vi "Stepper Motor.vi"() -> ()   [LabVIEW 2019]
doc: "The NI ELVIS III Custom FPGA Project template acquires button data from the onboard button and displays the button value on a Boolean indicator."
uses:
  <vilib>/Platform/TimedLoop/XDataNode/timing_clust.ctl
  <vilib>/Platform/TimedLoop/XDataNode/nitl_modes.ctl
  <vilib>/Platform/TimedLoop/XDataNode/wakeup.ctl
  <vilib>/Platform/TimedLoop/XDataNode/XDataNode.xnode
  <vilib>/Platform/TimedLoop/XDataNode/XDNodeRunTimeDep.lvlib
panel:
  in  "Microstep \nQuantization":dbl=100.0 format="%#_13g"
  in  "Step Period (ms)":i64(knob)=100 min=2 max=200 step=1 scale=2.0..200.0
  in  "Microstep Enable":bool
  out "Coil Activation":bool[](array[boolean])
  in  "Coil Activation Pattern":bool[][](array[boolean])
  out "Error Out":errorcluster
  in  "Stop Button":bool
  # "Mechatronic Actuators Board"
  # "Stepper Motor"
  # "A"
  # "B"
  # "C"
  # "D"
  # "A"
  # "B"
  # "C"
  # "D"
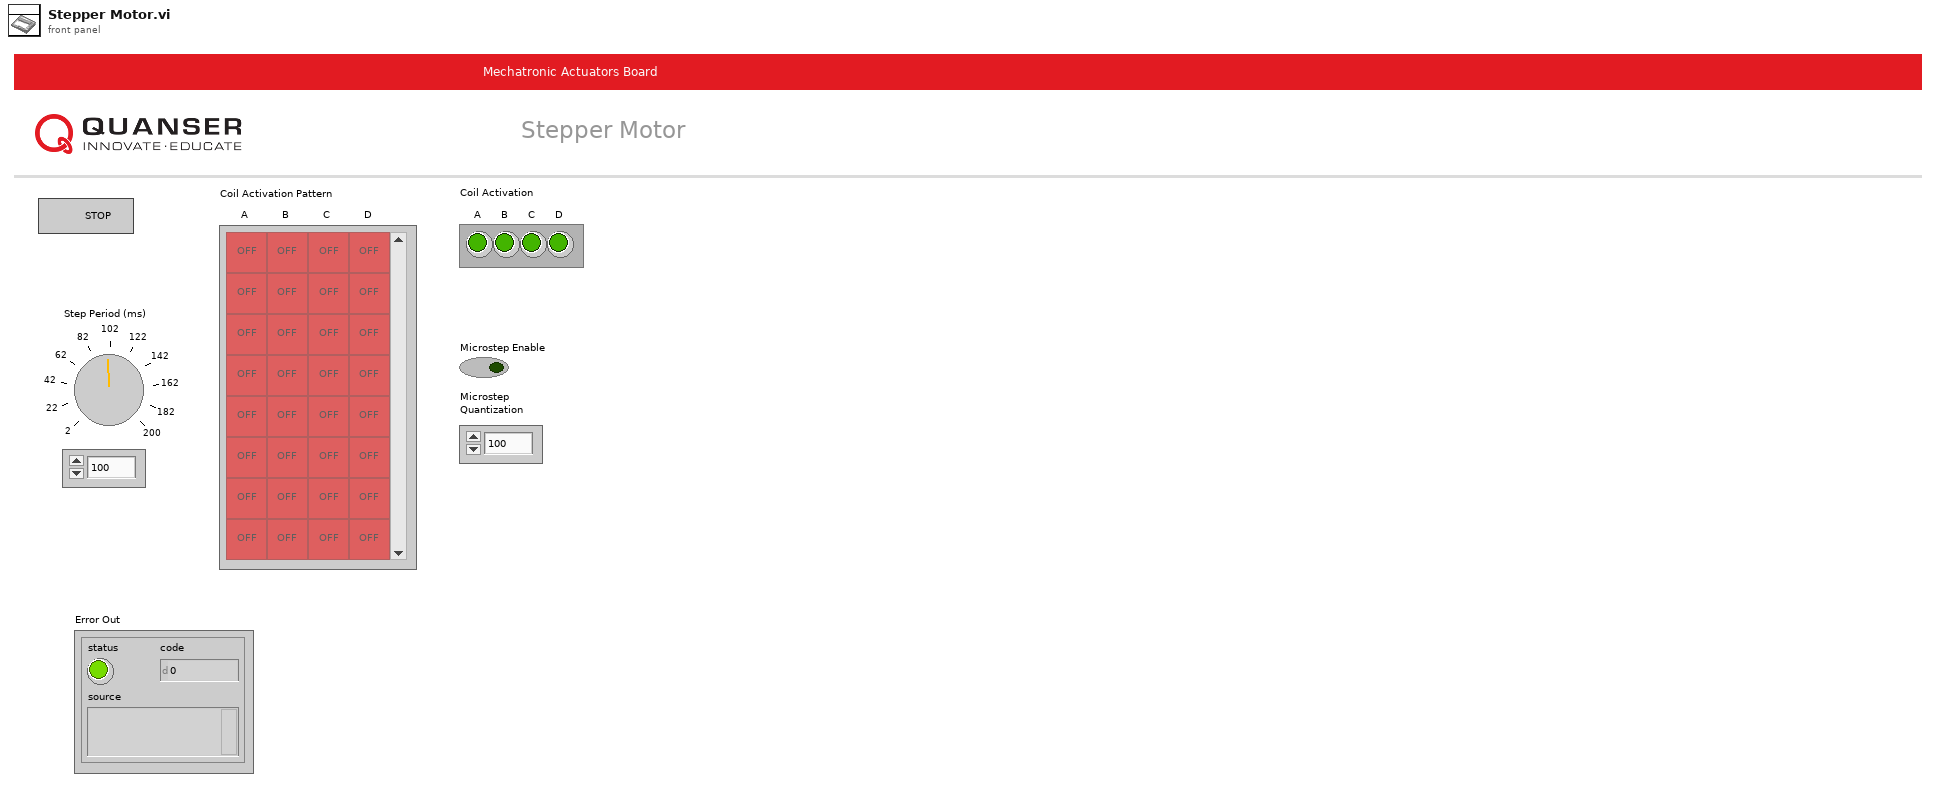
[diagram p1: front panel]
types:
  T1 = typedef "Actuators IO Cluster.ctl" = cluster{"Error":errorcluster, "FPGA Ref":refnum<k20>}
  T2 = typedef "XDNodeRunTimeDep.lvlib/timing_clust.ctl" = cluster{"Expected End [f-1]":u64, "Actual End [f-1]":u64, "Finished Late? [f-1]":bool, "Expected End [i-1]":u64, "Actual End [i-1]":u64, "Finished Late? [i-1]":bool, "Expected Start [i]":u64, "Actual Start [i]":u64, "Expected Start [f]":u64, "Actual Start [f]":u64, "Source Name":string, "Structure Name":string, "Period":i64, "Deadline":i64, "Offset":i64, "Start":i64, "Priority":i32, "Timeout":i32, "Mode":T3, "Wakeup Reason":T4, "Error":errorcluster, "Source Type":string, "Secondary Source Type":string, "Global End Time":u64, "Global Start Time":u64, "Frame Duration":u64, "Iteration Duration":u64, "Assigned CPU":i32, "I/O Scan Engine Mode":u32}
  T3 = typedef "XDNodeRunTimeDep.lvlib/nitl_modes.ctl" = enum32{"No Change", "Process missed periods, maintain original phase", "Discard missed periods, maintain original phase", "Process missed periods, ignore original phase", "Discard missed periods, ignore original phase"}
  T4 = typedef "XDNodeRunTimeDep.lvlib/wakeup.ctl" = enum32{"Normal", "Aborted", "Asynchronous wakeup", "Timing source error", "Timed loop error", "Timeout"}
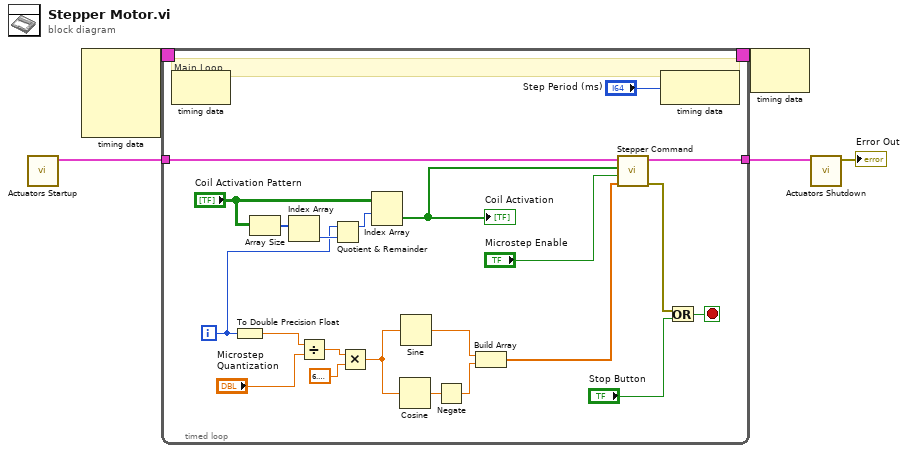
[diagram p0: block diagram]
diagram:
  n1 = call "Actuators Startup.vi"() -> ("IO Cluster OUT"=w3:T1)  [unwired: 11 in]
  n2 = node-c288() -> (w5:T2)  [unwired: 4 in]
  n3 = timed-loop {
    timing: w5 -> [_]
    timing-out: [_] -> w4
    tunnel: w3 -> [w25]
    tunnel: [w24] -> w2
    i -> [w13]
    stop <- w27 stop-if-true
    # "Main Loop"
    n4 = node-c288() -> ()  [unwired: 1 in, 1 out]
    n5 = To Double Precision Float(number=w13) -> (double precision float=w11:dbl)
    n6 = Array Size(array="Coil Activation Pattern") -> (size(s)=w22:i32[])
    n7 = Index Array(array=w22) -> (element=w19:i32)  [unwired: 1 in]
    n8 = Divide(x=w11, y="Microstep \nQuantization") -> (x/y=w9:dbl)
    n9 = Quotient & Remainder(x=w13, y=w19) -> (x-y*floor(x/y)=w20:i32)  [unwired: 1 out]
    n10 = Multiply(x=w9, y=6.283185307179586) -> (x*y=w10:dbl)
    n11 = Index Array(array="Coil Activation Pattern", index (row)=w20) -> (element=w18:bool[])  [unwired: 1 in]
    "Coil Activation" <- w18
    n12 = Cosine(x=w10) -> (cos(x)=w7:dbl)
    n13 = Sine(x=w10) -> (sin(x)=w16:dbl)
    n14 = Negate(x=w7) -> (-x=w6:dbl)
    n15 = Build Array(w16, w6) -> (w15:dbl[])
    n16 = call "Stepper Command.vi"("Microstep Coil Activation"=w15, "Microstep Enable"="Microstep Enable", "Stepper Coil Activation"=w18, "IO Cluster IN"=w25) -> ("Error Out"=w23:errorcluster, "IO Cluster OUT"=w24:T1)  [unwired: 6 in]
    n17 = node-c288("Step Period (ms)") -> ()  [unwired: 1 out]
    n18 = Or(x=w23, y="Stop Button") -> (x .or. y?=w27:bool)
  }
  n19 = node-c288(w4) -> ()  [unwired: 1 out]
  n20 = call "Actuators Shutdown.vi"("IO Cluster IN"=w2) -> ("Error Out"=→"Error Out":errorcluster)  [unwired: 10 in]
